vi "Remove Quotes.vi"(1 "String":string) -> (0 "String without Quotes":string)   [LabVIEW 2013, in "LV JSON.lvlib"]
doc: "Removes double quotes from beginning and end of string. Ignores quotes in-between."
uses:
  LV JSON.lvlib
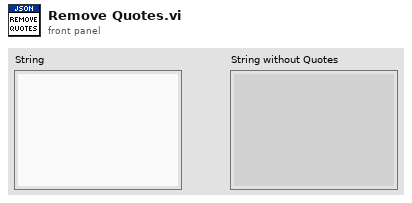
[diagram p1: front panel]
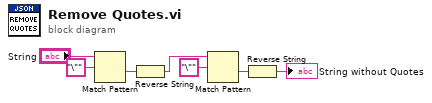
[diagram p0: block diagram]
diagram:
  n1 = Match Pattern(string="String", regular expression="\"") -> (after substring=w5:string)  [unwired: 1 in, 3 out]
  n2 = Reverse String(1:w5) -> (0:w3:string)
  n3 = Match Pattern(string=w3, regular expression="\"") -> (after substring=w2:string)  [unwired: 1 in, 3 out]
  n4 = Reverse String(1:w2) -> (0:→"String without Quotes":string)
